vi "Sort Channel Data.vi"(0 "Key":enum16{"SimTC", "Calibration", "VO", "CO"}[](array[ring]), 5 "Input Data":dbl[](array[numeric]), 11 "error in (no error)":errorcluster) -> (4 "VO Channels":dbl[](array[numeric]), 6 "CO Channels":dbl[](array[numeric]), 8 "SimTC Channels":dbl[](array[numeric]), 10 "Calibration Channels":dbl[](array[numeric]), 15 "error out":errorcluster)   [LabVIEW 2011, in "Simulated Thermocouple Custom Device.lvlib"]
uses:
  Simulated Thermocouple Custom Device.lvlib
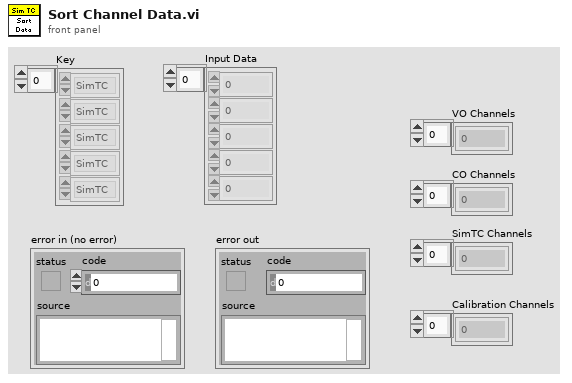
[diagram p1: front panel]
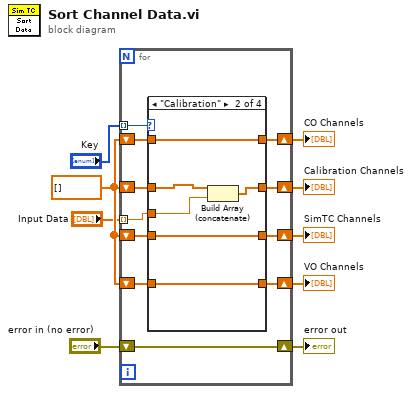
[diagram p0: block diagram]
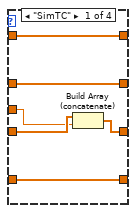
[diagram p2: hidden frame]
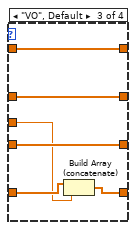
[diagram p3: hidden frame]
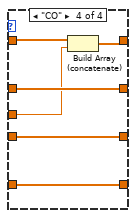
[diagram p4: hidden frame]
diagram:
  w9 = dbl[] []
  n1 = for {
    tunnel: "Key" -> [w20] mode=indexing
    shift-right: [w10] -> w7
    shift-left: "error in (no error)" -> [w10]
    tunnel: "Input Data" -> [w15] mode=indexing
    shift-right: [w14] -> w4
    shift-left: w9 -> [w19]
    shift-right: [w13] -> w3
    shift-left: w9 -> [w18]
    shift-right: [w12] -> w2
    shift-left: w9 -> [w17]
    shift-right: [w11] -> w1
    shift-left: w9 -> [w16]
    n2 = case shown="\"Calibration\"" w20 {
      tunnel: w19 -> [w26 w30 w34 w44]
      tunnel: w18 -> [w25 w31 w38 w40]
      tunnel: w17 -> [w22 w32 w37 w43]
      tunnel: w16 -> [w24 w28 w36 w42]
      tunnel: w15 -> [w21 w27 w33 w39]
      tunnel: [w26 w30 w35 w44] -> w14
      tunnel: [w25 w31 w38 w41] -> w13
      tunnel: [w23 w32 w37 w43] -> w12
      tunnel: [w24 w29 w36 w42] -> w11
      frame "SimTC" {
        n3 = Build Array (concatenate)(w22, w21) -> (w23:dbl[])
      }
      frame "Calibration" {
        n4 = Build Array (concatenate)(w28, w27) -> (w29:dbl[])
      }
      frame "VO", Default {
        n5 = Build Array (concatenate)(w34, w33) -> (w35:dbl[])
      }
      frame "CO" {
        n6 = Build Array (concatenate)(w40, w39) -> (w41:dbl[])
      }
    }
  }
  "error out" <- w7
  "VO Channels" <- w4
  "CO Channels" <- w3
  "SimTC Channels" <- w2
  "Calibration Channels" <- w1
